vi "svx_SC Line CheckboxToIndex.vi"(4 "All Children Tags":string[](array[string]), 10 "Coords":T1, 11 "Tree ref in":refnum<vi>) -> (0 "State Changed?":bool, 2 "index":i32[](array[numeric]), 3 "Tree ref out":refnum<vi>)   [LabVIEW 2017, in "SVX SC Line.xctl"]
uses:
  <vilib>/addons/_XControls/Shaft Centerline/SVX SC Line.xctl
  <vilib>/Utility/miscctls.llb/LVPoint32TypeDef.ctl
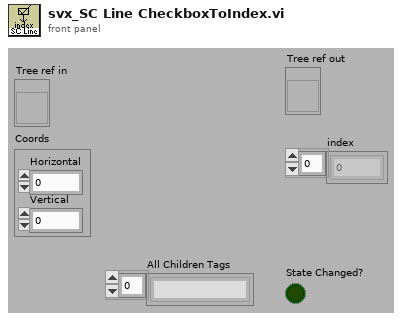
[diagram p1: front panel]
types:
  T1 = typedef "LVPoint32TypeDef.ctl" = cluster{"Horizontal":i32, "Vertical":i32}
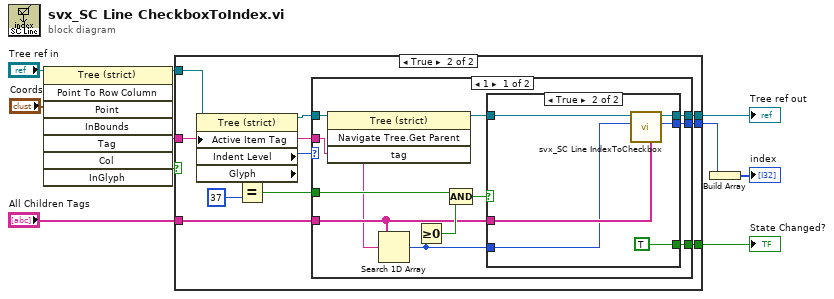
[diagram p0: block diagram]
diagram:
  n1 = invoke on="Invoke Node" class="Tree (strict)" method="Point To Row Column"(reference="Tree ref in", "Point"="Coords") -> (reference out=w10:refnum<vi>, "Tag"=w9:string, "InGlyph"=w8:bool)  [unwired: 6 in, 5 out]
  n2 = case shown="True" w8 {
    tunnel: w10 -> [w11 w22]
    tunnel: w9 -> [_ w20]
    tunnel: "All Children Tags" -> [_ w16]
    tunnel: [_ w14] -> w2
    tunnel: [w11 w13] -> w5
    tunnel: [_ w12] -> w4
    frame False {
    }
    frame True {
      n3 = property class="Tree (strict)"(reference=w22, "Active Item Tag"=w20) -> (reference out=w21:refnum<vi>, "Indent Level"=w18:i32, "Glyph"=w17:i32)  [unwired: 1 in, 1 out]
      n4 = Equal?(x=w17, y=37) -> (x = y?=w15:bool)
      n5 = case shown="1" w18 {
        tunnel: w21 -> [w33 w40]
        tunnel: w20 -> [w24 _]
        tunnel: w16 -> [w29 _]
        tunnel: w15 -> [w30 _]
        tunnel: [w27 _] -> w14
        tunnel: [w26 w40] -> w13
        tunnel: [w25 _] -> w12
        frame 1 {
          n6 = invoke on="Invoke Node" class="Tree (strict)" method="Navigate Tree.Get Parent"(reference=w33, "tag"=w24) -> (reference out=w31:refnum<vi>)  [unwired: 2 in, 3 out]
          n7 = Search 1D Array(1D array=w29, element=w24) -> (index of element=w23:i32)  [unwired: 1 in]
          n8 = Greater Or Equal To 0?(x=w23) -> (x >= 0?=w32:bool)
          n9 = Compound Arithmetic op=AND(w30, w32) -> (w28:bool)
          n10 = case shown="True" w28 {
            tunnel: w31 -> [w34 w39]
            tunnel: w29 -> [_ w38]
            tunnel: [_ w35] -> w27
            tunnel: [w34 w37] -> w26
            tunnel: [_ TRUE ("State Changed?")] -> w25
            tunnel: w23 -> [_ w35]
            frame False {
            }
            frame True {
              n11 = call <vilib>:"svx_SC Line IndexToCheckbox.vi"("All Children Tags"=w38, "RowIdx"=w35, "Tree ref in"=w39) -> ("Tree ref out"=w37:refnum<vi>)  [unwired: 8 in]
            }
          }
        }
        frame Default {
        }
      }
    }
  }
  "Tree ref out" <- w5
  "State Changed?" <- w4
  n12 = Build Array(w2) -> (→"index":i32[])
